vi "Close-TCP.vi"(8 "error in (no error)":errorcluster, 11 "SM1000-control in":T1) -> (0 "error out":errorcluster, 1 "Succes?":bool, 3 "SM1000-control out":T1)   [LabVIEW 2013, in "SLMControl.lvlib" / "SM1000.lvclass"]
uses:
  SM1000.lvclass
  Object-reference.ctl
  SM1000.lvclass/SM1000.ctl
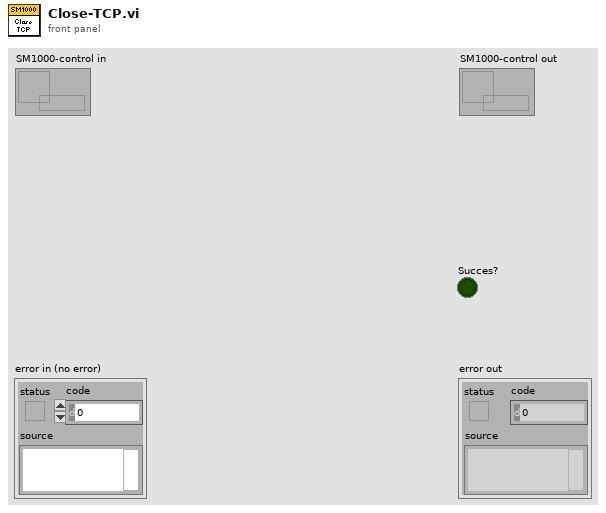
[diagram p1: front panel]
types:
  T1 = typedef "SLMControl.lvlib/SM1000.lvclass/Object-reference.ctl" = refnum<data-value>
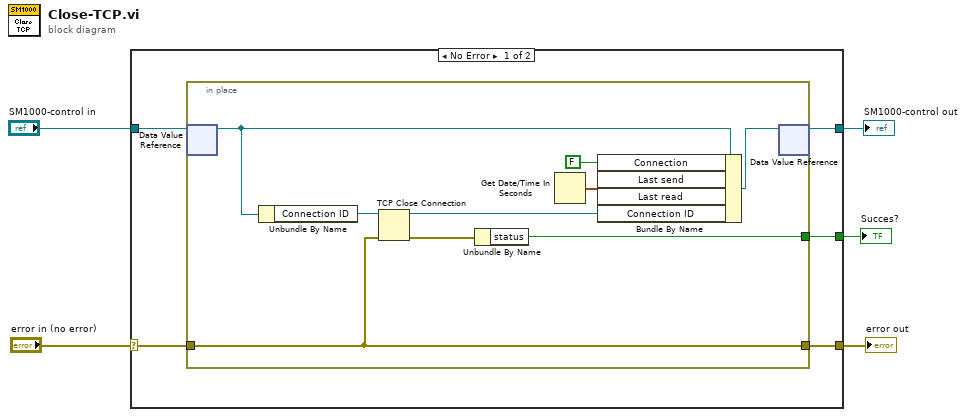
[diagram p0: block diagram]
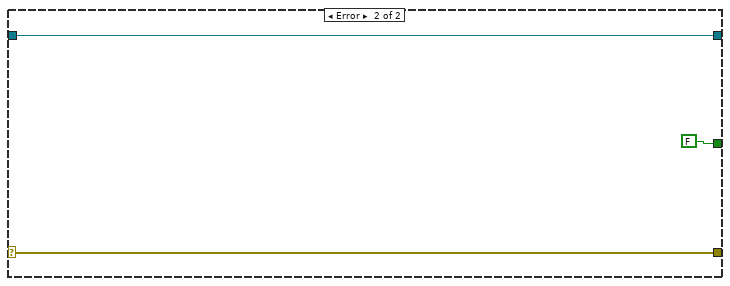
[diagram p2: hidden frame]
diagram:
  n1 = case shown="No Error" "error in (no error)" {
    selector: "error in (no error)" -> [w8 w22]
    tunnel: [w7 w22] -> w4
    tunnel: [w9 w21] -> w2
    tunnel: "SM1000-control in" -> [w10 w21]
    tunnel: [w6 FALSE] -> w1
    frame No Error {
      n2 = in-place {
        in-place-border: w8 -> [w13]
        in-place-border: [w13] -> w7
        in-place-border: [w11] -> w6
        n3 = in-place-dvr #1(w10) -> (w19:refnum<class "SM1000.lvclass">)  [unwired: 1 out]
        n4 = Unbundle By Name(w19) -> ("Connection ID"=w15:refnum<k5>)
        n5 = TCP Close Connection(connection ID=w15, error in (no error)=w13) -> (connection ID out=w18:refnum<k5>, error out=w14:errorcluster)  [unwired: 1 in]
        n6 = Unbundle By Name(w14) -> ("status"=w11:bool)
        n7 = Get Date/Time In Seconds() -> (seconds since 1Jan1904=w17:timestamp)
        n8 = Bundle By Name(cluster=w19, "Connection"=FALSE ("TCP status.Connection"), "Last send"=w17, "Last read"=w17, "Connection ID"=w18) -> (w16:refnum<class "SM1000.lvclass">)
        n9 = in-place-dvr #1(w16) -> (w9:T1)  [unwired: 1 out]
      }
    }
    frame Error {
    }
  }
  "error out" <- w4
  "SM1000-control out" <- w2
  "Succes?" <- w1
